vi "Bolean Array to String.vi"(11 "Bolean Array":bool[](array[boolean])) -> (3 "Bolean String":string)   [LabVIEW 2021]
panel:
  # "Bolean Array to String\n2015-06-12 17:19:41\n蒋松"
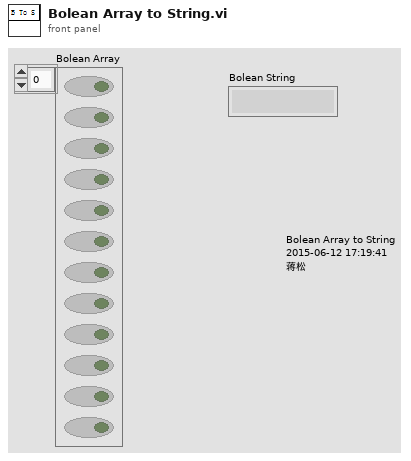
[diagram p1: front panel]
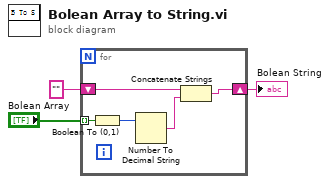
[diagram p0: block diagram]
diagram:
  n1 = for {
    tunnel: "Bolean Array" -> [w8] mode=indexing
    shift-right: [w4] -> w1
    shift-left: "" -> [w6]
    n2 = Boolean To (0,1)(Boolean=w8) -> (0, 1=w7:i16)
    n3 = Number To Decimal String(number=w7) -> (decimal integer string=w5:string)  [unwired: 1 in]
    n4 = Concatenate Strings(w6, w5) -> (w4:string)
  }
  "Bolean String" <- w1
